vi "P3.7.vi"() -> ()   [LabVIEW 2020]
uses:
  <vilib>/Analysis/2dsp.llb/1D Convolution (DBL).vi
  <vilib>/Analysis/NI_AALPro.lvlib
panel:
  out "DFT X2":dbl[](graph)
  out "DFT X1":dbl[](graph)
  out "X * Y - temporal":dbl[](graph)
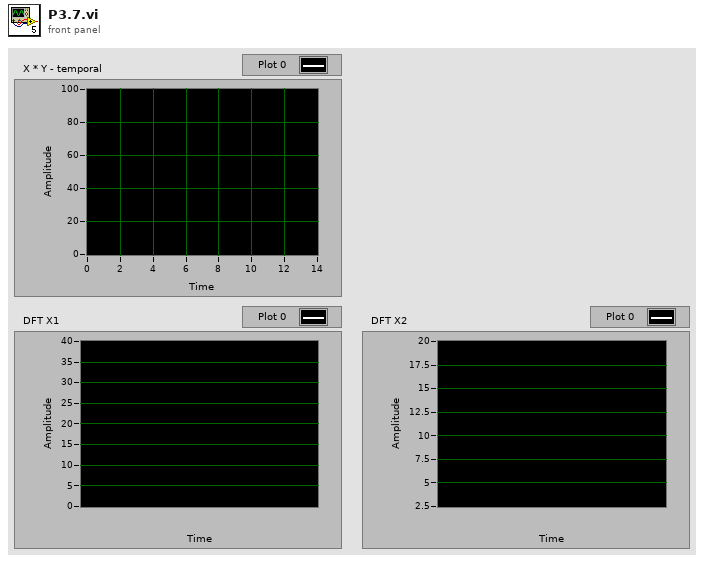
[diagram p1: front panel]
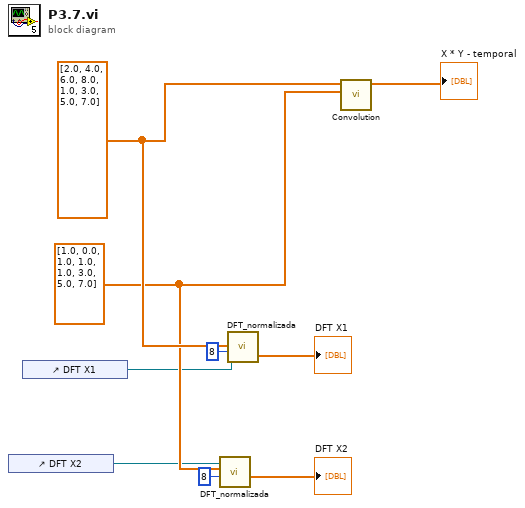
[diagram p0: block diagram]
diagram:
  w7 = dbl[] [1.0, 0.0, 1.0, 1.0, 1.0, 3.0, 5.0, 7.0]
  w8 = dbl[] [2.0, 4.0, 6.0, 8.0, 1.0, 3.0, 5.0, 7.0]
  n1 = control-ref of="DFT X2"() -> (w1:refnum<vi>)
  n2 = control-ref of="DFT X1"() -> (w2:refnum<vi>)
  n3 = call "DFT_normalizada.vi"("FFT size"=8, "X[n]"=w7, "WaveformGraph in"=w1) -> ("DFTnorm"=→"DFT X2":cdb[])  [unwired: 8 in]
  n4 = call "DFT_normalizada.vi"("FFT size"=8, "X[n]"=w8, "WaveformGraph in"=w2) -> ("DFTnorm"=→"DFT X1":cdb[])  [unwired: 8 in]
  n5 = call-poly <vilib>:"Convolution.vi"("Y"=w7, "X"=w8) -> ("X * Y"=→"X * Y - temporal":dbl[])  [unwired: 8 in, 1 out]
